vi "ReadConfigConectionSubVI.vi"(3 "error in (no error)":errorcluster, 4 "dup path":path, 5 "Conections in":T1) -> (0 "error out":errorcluster, 1 "section names":string[](array[string]), 2 "Conections out":T1)   [LabVIEW 2016]
doc: "Reads the config file and returns the conections and <b>section names</b> of the file."
uses:
  <vilib>/Utility/config.llb/Read Key (String).vi
  <vilib>/Utility/config.llb/NI_LVConfig.lvlib
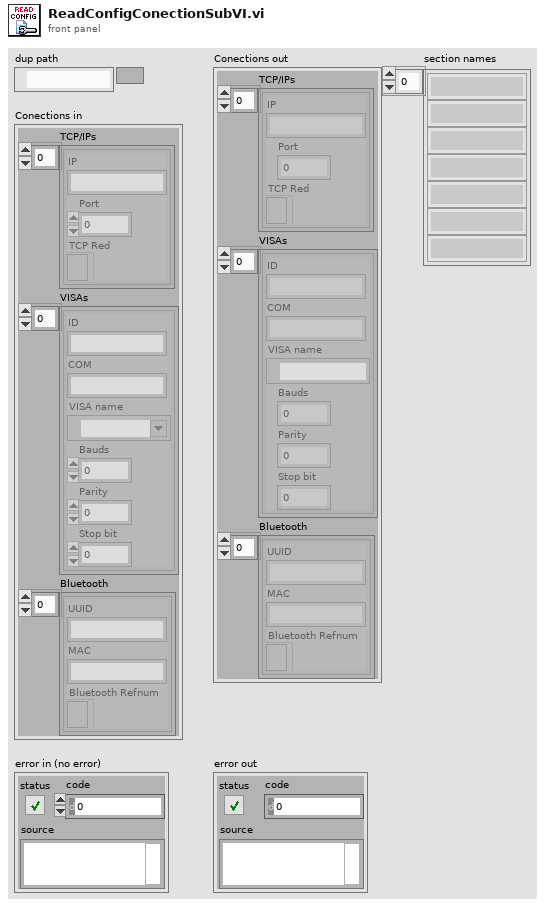
[diagram p1: front panel]
types:
  T1 = cluster{"TCP/IPs":cluster{"IP":string, "Port":u16, "TCP Red":refnum<k5>}[], "VISAs":cluster{"ID":string, "COM":string, "VISA name":refnum<visa-resource-name>, "Bauds":dbl, "Parity":u16, "Stop bit":u16}[], "Bluetooth":cluster{"UUID":string, "MAC":string, "Bluetooth Refnum":refnum<k31>}[]}
  T2 = typedef "NI_LVConfig.lvlib/Config Data RefNum.ctl" = refnum<k1>
  T3 = cluster{"ID":string, "COM":string, "VISA name":refnum<visa-resource-name>, "Bauds":dbl, "Parity":u16, "Stop bit":u16}[]
  T4 = cluster{"ID":string, "COM":string, "VISA name":refnum<visa-resource-name>, "Bauds":dbl, "Parity":u16, "Stop bit":u16}
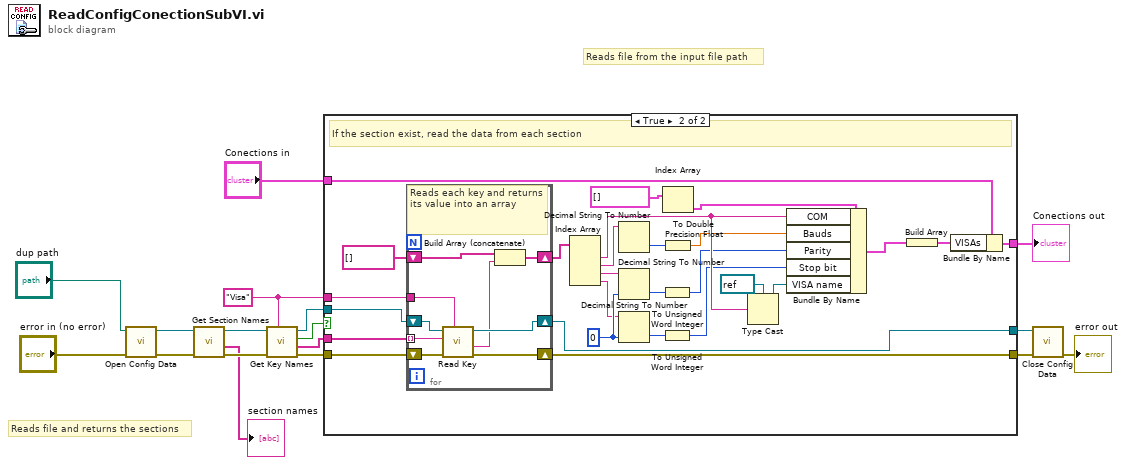
[diagram p0: block diagram]
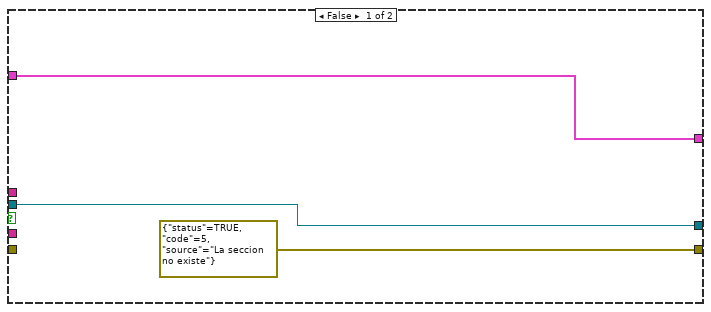
[diagram p2: hidden frame]
diagram:
  w14 = "Visa" ("section")
  # "Reads file and returns the sections"
  # "Reads file from the input file path"
  n1 = call <vilib>:"Open Config Data.vi"("error in (no error)"="error in (no error)", "configuration file path"="dup path") -> ("error out"=w4:errorcluster, "refnum"=w5:T2)  [unwired: 7 in, 1 out]
  n2 = call <vilib>:"Get Section Names.vi"("error in (no error)"=w4, "refnum"=w5) -> ("error out"=w3:errorcluster, "section names"=→"section names":string[], "refnum out"=w2:T2)  [unwired: 7 in]
  n3 = call <vilib>:"Get Key Names.vi"("section"=w14, "error in (no error)"=w3, "refnum"=w2) -> ("error out"=w12:errorcluster, "key names"=w15:string[], "section exists?"=w11:bool, "refnum out"=w13:T2)  [unwired: 5 in]
  n4 = case shown="True" w11 {
    tunnel: [errorcluster {"status"=TRUE, "code"=5, "source"="La seccion no existe"} ("error out") w38] -> w6
    tunnel: [w20 w47] -> w8
    tunnel: "Conections in" -> [w19 w46]
    tunnel: [w19 w45] -> w10
    tunnel: w12 -> [_ w44]
    tunnel: w13 -> [w20 w43]
    tunnel: w14 -> [_ w42]
    tunnel: w15 -> [_ w41]
    frame False {
    }
    frame True {
      w33 = 0
      # "If the section exist, read the data from each section"
      n5 = for {
        shift-right: [w54] -> w38
        shift-left: w44 -> [w56]
        shift-right: [w53] -> w47
        shift-left: w43 -> [w55]
        tunnel: w42 -> [w52]
        tunnel: w41 -> [w51] mode=indexing
        shift-right: [w49] -> w24
        shift-left: string[] [] -> [w50]
        # "Reads each key and returns its value into an array"
        n6 = call-poly <vilib>:"Read Key.vi"("section"=w52, "error in (no error)"=w56, "key"=w51, "refnum"=w55) -> ("error out"=w54:errorcluster, "value"=w48:string, "refnum out"=w53:T2)  [unwired: 4 in, 1 out]
        n7 = Build Array (concatenate)(w50, w48) -> (w49:string[])
      }
      n8 = Index Array(array=w24) -> (element #1=w39:string, element #2=w28:string, element #3=w29:string, element #4=w30:string)  [unwired: 4 in]
      n9 = Decimal String To Number(string=w28) -> (number=w31:i32)  [unwired: 2 in, 1 out]
      n10 = Decimal String To Number(string=w29, default (0L)=w33) -> (number=w34:i32)  [unwired: 1 in, 1 out]
      n11 = Decimal String To Number(string=w30, default (0L)=w33) -> (number=w36:i32)  [unwired: 1 in, 1 out]
      n12 = To Unsigned Word Integer(number=w34) -> (unsigned 16bit integer=w35:u16)
      n13 = To Unsigned Word Integer(number=w36) -> (unsigned 16bit integer=w37:u16)
      n14 = Index Array(array=T3 [] ("VISAs")) -> (element=w26:T4)  [unwired: 1 in]
      n15 = To Double Precision Float(number=w31) -> (double precision float=w32:dbl)
      n16 = Type Cast(type=refnum<visa-resource-name> refnum ("VISA name"), x=w39) -> (*(type *) &x=w21:refnum<visa-resource-name>)
      n17 = Bundle By Name(cluster=w26, "COM"=w39, "Bauds"=w32, "Parity"=w35, "Stop bit"=w37, "VISA name"=w21) -> (w25:T4)
      n18 = Build Array(w25) -> (w23:T3)
      n19 = Bundle By Name(cluster=w46, "VISAs"=w23) -> (w45:T1)
    }
  }
  "Conections out" <- w10
  n20 = call <vilib>:"Close Config Data.vi"("error in (no error)"=w6, "refnum"=w8) -> ("error out"=→"error out":errorcluster)  [unwired: 8 in, 1 out]
